vi "ID Query.vi"(0 "VISA resource name":refnum<visa-resource-name>, 5 "error in":errorcluster) -> (14 "VISA resource name out":refnum<visa-resource-name>, 15 "Manufacturer":string, 16 "Model Name":string, 17 "Serial Number":i32, 18 "Firmware Revision":string, 19 "error out":errorcluster)   [LabVIEW 2019, in "Andeen-Hagerling 2700(400 firmware).lvlib"]
doc: "Reports the manufacturer, model, serial number and firmware version."
uses:
  Andeen-Hagerling 2700(400 firmware).lvlib
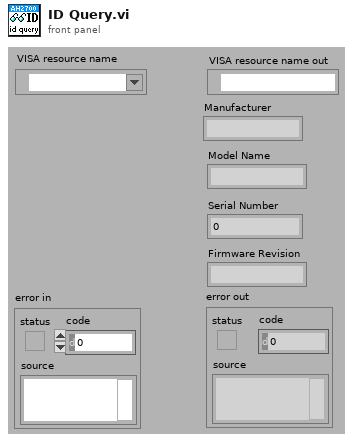
[diagram p1: front panel]
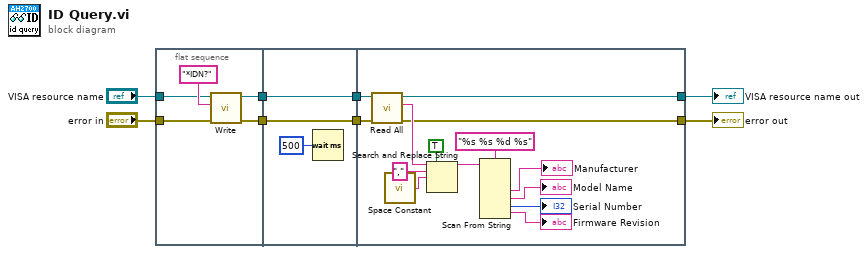
[diagram p0: block diagram]
diagram:
  n1 = flat-sequence {
    tunnel: "VISA resource name" -> [w12]
    tunnel: "error in" -> [w11]
    tunnel: [w10] -> w8
    tunnel: [w9] -> w7
    tunnel: w8 -> [w14]
    tunnel: w7 -> [w15]
    tunnel: [w15] -> w6
    tunnel: [w14] -> w5
    tunnel: w6 -> [w29]
    tunnel: w5 -> [w30]
    tunnel: [w18] -> w1
    tunnel: [w17] -> w2
    frame #0 {
      n2 = call "Write.vi"("error in"=w11, "command"="*IDN?", "VISA resource name"=w12) -> ("error out"=w9:errorcluster, "VISA resource name out"=w10:refnum<visa-resource-name>)  [unwired: 7 in]
    }
    frame #1 {
      n3 = Wait (ms)(milliseconds to wait=u32 500) -> ()  [unwired: 1 out]
    }
    frame #2 {
      n4 = call "Read All.vi"("error in"=w29, "VISA resource name"=w30) -> ("error out"=w17:errorcluster, "Message"=w19:string, "VISA resource name out"=w18:refnum<visa-resource-name>)  [unwired: 7 in]
      n5 = call <vilib>:"Space Constant.vi"() -> ("String"=w23:string)
      n6 = Search and Replace String(replace all?=TRUE ("replace all? (F)"), input string=w19, search string=",", replace string=w23) -> (result string=w24:string)  [unwired: 4 in, 3 out]
      n7 = Scan From String(format string="%s %s %d %s", input string=w24) -> (output 1=→"Manufacturer":string, output 2=→"Model Name":string, output 3=→"Serial Number":i32, output 4=→"Firmware Revision":string)  [unwired: 6 in, 3 out]
    }
  }
  "VISA resource name out" <- w1
  "error out" <- w2
